vi "U-sonic range finder (Host).vi"() -> ()   [LabVIEW 2013]
uses:
  <vilib>/Platform/TimedLoop/XDataNode/timing_clust.ctl
  <vilib>/Platform/TimedLoop/XDataNode/nitl_modes.ctl
  <vilib>/Platform/TimedLoop/XDataNode/wakeup.ctl
  <vilib>/rvi/interface/common/niFpgaWaitOnOcc.vi
  <vilib>/FPGAPlugInAG/myRIO-1900/niLvFpga_Open_myRIO-1900.vi
  <vilib>/rvi/interface/common/dynamic/niFpgaDynamicAddResources.vi
  <vilib>/Utility/error.llb/Error Cluster From Error Code.vi
  <vilib>/rvi/errors/niLvFpgaAdjustHostInterfaceError.vi
  <vilib>/FPGAPlugInAG/Dynamic/niLvFpga_Close_Dynamic.vi
  <vilib>/Platform/TimedLoop/XDataNode/XDataNode.xnode
  <vilib>/rvi/interface/nirviOpenFPGA/nirviOpenFPGA.xnode
  New folder/FPGA Bitfiles/1-wireinterface_FPGATarget_Ultrasonicrangef_6rkNm1IqGok.lvbitx
  Ultrasonic_range_finder.vi
  <vilib>/rvi/interface/nirviReadWriteControl/nirviReadWriteControl.xnode
  <vilib>/rvi/interface/nirviCloseFPGA/nirviCloseFPGA.xnode
  <vilib>/Platform/TimedLoop/XDataNode/XDNodeRunTimeDep.lvlib
  NiFpgaLv.dll
  <vilib>/rvi/interface/Simulation/niFpgaSimulationCallBeginRW.vi
panel:
  out "error out":errorcluster
  out "C/DIO2":bool
  in  "CM or INCH":bool
  out "Measured Pulse Width (usec)":dbl format="%0.9f"
  out "Distance":dbl format="%0.9f"
  in  "stop":bool
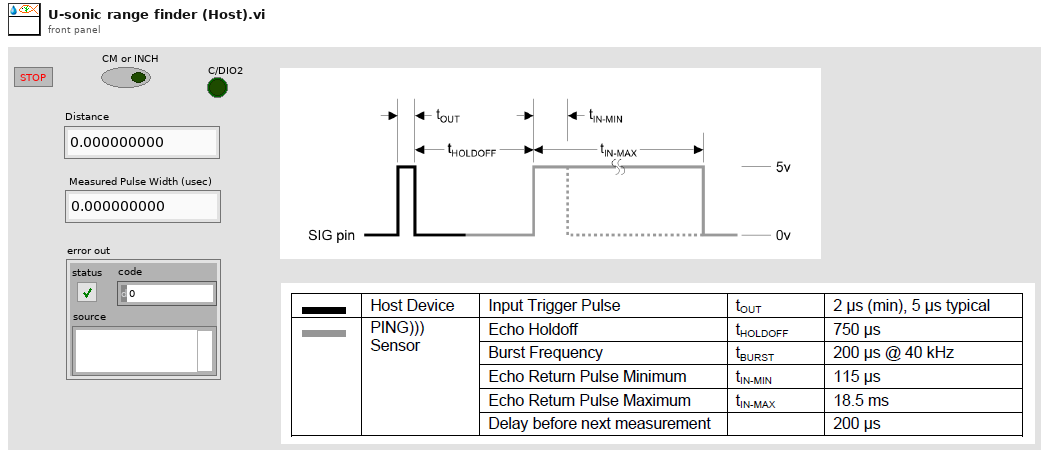
[diagram p1: front panel]
types:
  T1 = typedef "XDNodeRunTimeDep.lvlib/timing_clust.ctl" = cluster{"Expected End [f-1]":u64, "Actual End [f-1]":u64, "Finished Late? [f-1]":bool, "Expected End [i-1]":u64, "Actual End [i-1]":u64, "Finished Late? [i-1]":bool, "Expected Start [i]":u64, "Actual Start [i]":u64, "Expected Start [f]":u64, "Actual Start [f]":u64, "Source Name":string, "Structure Name":string, "Period":i64, "Deadline":i64, "Offset":i64, "Start":i64, "Priority":i32, "Timeout":i32, "Mode":T2, "Wakeup Reason":T3, "Error":errorcluster, "Source Type":string, "Secondary Source Type":string, "Global End Time":u64, "Global Start Time":u64, "Frame Duration":u64, "Iteration Duration":u64, "Assigned CPU":i32, "I/O Scan Engine Mode":u32}
  T2 = typedef "XDNodeRunTimeDep.lvlib/nitl_modes.ctl" = enum32{"No Change", "Process missed periods, maintain original phase", "Discard missed periods, maintain original phase", "Process missed periods, ignore original phase", "Discard missed periods, ignore original phase"}
  T3 = typedef "XDNodeRunTimeDep.lvlib/wakeup.ctl" = enum32{"Normal", "Aborted", "Asynchronous wakeup", "Timing source error", "Timed loop error", "Timeout"}
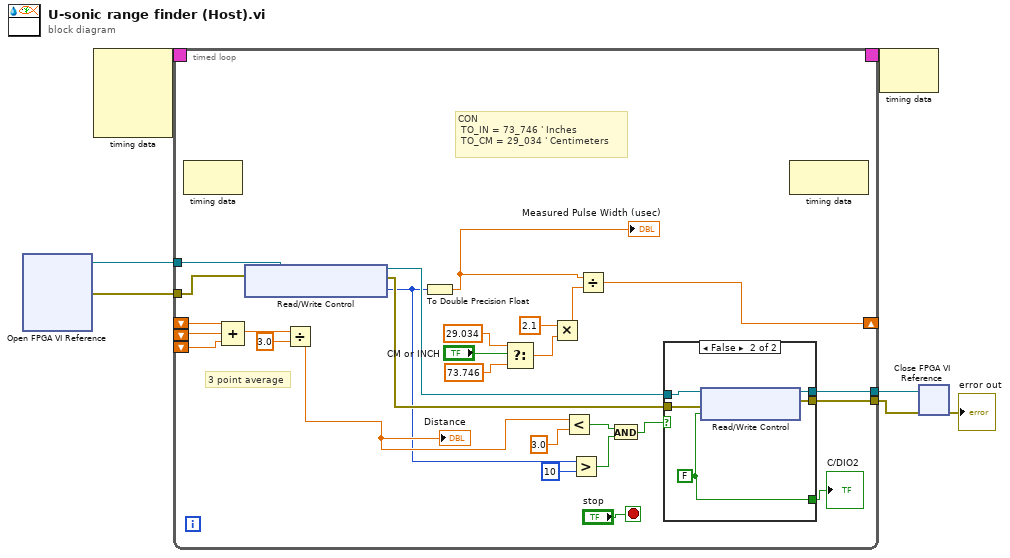
[diagram p0: block diagram]
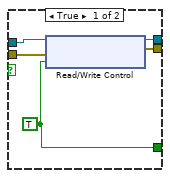
[diagram p2: hidden frame]
diagram:
  n1 = xnode "Open FPGA VI Reference"() -> ("FPGA VI Reference Out"=w5:refnum<k20>, "error out"=w4:errorcluster)  [unwired: 2 in]
  n2 = node-c288() -> (w7:T1)  [unwired: 4 in]
  n3 = timed-loop {
    timing: w7 -> [_]
    timing-out: [_] -> w6
    tunnel: w5 -> [w34]
    tunnel: w4 -> [w33]
    shift-right: [w25] -> _
    shift-left: _ -> [w24]
    shift-left: _ -> [w23]
    shift-left: _ -> [w22]
    tunnel: [w14] -> w3
    tunnel: [w13] -> w2
    stop <- "stop" stop-if-true
    # "3 point average"
    # "CON \n TO_IN = 73_746 ' Inches \n TO_CM = 29_034 ' Centimeters"
    n4 = node-c288() -> ()  [unwired: 1 in, 1 out]
    n5 = Compound Arithmetic op=ADD(w24, w23, w22) -> (w21:dbl)
    n6 = xnode "Read/Write Control"("FPGA VI Reference In"=w34, "error in"=w33) -> ("FPGA VI Reference Out"=w16:refnum<k20>, "error out"=w15:errorcluster, "Measured Period (usec)"=w10:u32)
    n7 = Divide(x=w21, y=3.0) -> (x/y=w19:dbl)
    "Distance" <- w19
    n8 = To Double Precision Float(number=w10) -> (double precision float=w32:dbl)
    "Measured Pulse Width (usec)" <- w32
    n9 = Select(t=29.034 ("x"), s="CM or INCH", f=73.746 ("x")) -> (s? t:f=w27:dbl)
    n10 = Multiply(x=2.1, y=w27) -> (x*y=w26:dbl)
    n11 = Less?(x=w19, y=3.0) -> (x < y?=w11:bool)
    n12 = Greater?(x=w10, y=u32 10) -> (0:w8:bool)
    n13 = Divide(x=w32, y=w26) -> (x/y=w25:dbl)
    n14 = And(x=w11, y=w8) -> (x .and. y?=w12:bool)
    n15 = case shown="False" w12 {
      tunnel: [w36 w41] -> w17
      tunnel: w16 -> [w40 w45]
      tunnel: w15 -> [w39 w44]
      tunnel: [w38 w43] -> w14
      tunnel: [w37 w42] -> w13
      frame True {
        w36 = TRUE ("C/DIO2")
        n16 = xnode "Read/Write Control"("FPGA VI Reference In"=w40, "error in"=w39, "Control On/Off"=w36) -> ("FPGA VI Reference Out"=w38:refnum<k20>, "error out"=w37:errorcluster)
      }
      frame False {
        w41 = FALSE ("C/DIO2")
        n17 = xnode "Read/Write Control"("FPGA VI Reference In"=w45, "error in"=w44, "Control On/Off"=w41) -> ("FPGA VI Reference Out"=w43:refnum<k20>, "error out"=w42:errorcluster)
      }
    }
    "C/DIO2" <- w17
    n18 = node-c288() -> ()  [unwired: 1 in, 1 out]
  }
  n19 = node-c288(w6) -> ()  [unwired: 1 out]
  n20 = xnode "Close FPGA VI Reference"("FPGA VI Reference In"=w3, "error in"=w2) -> ("error out"=→"error out":errorcluster)
